vi "Precission to 3 digits.vi"(8 "error in":errorcluster, 11 "Numeric":dbl format="%#_13g") -> (0 "error out":errorcluster, 3 "number":dbl)   [LabVIEW 2015]
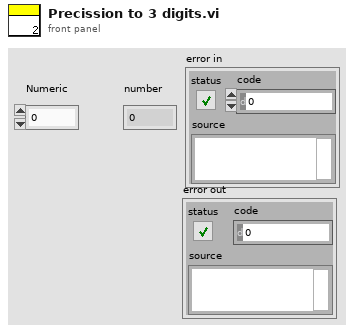
[diagram p1: front panel]
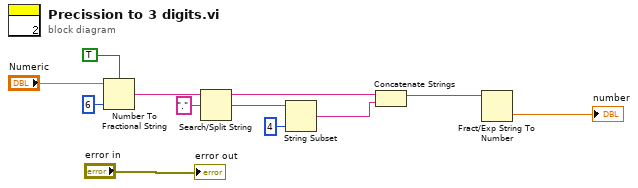
[diagram p0: block diagram]
diagram:
  n1 = Number To Fractional String(use system decimal point (T)=TRUE, number="Numeric", precision (6)=i16 6) -> (F-format string=w5:string)  [unwired: 1 in]
  n2 = Search/Split String(string=w5, search string/char (-)=".") -> (substring before match=w10:string, match + rest of string=w7:string)  [unwired: 1 in, 1 out]
  n3 = String Subset(string=w7, length (rest)=4 ("length (rest)")) -> (substring=w9:string)  [unwired: 1 in]
  n4 = Concatenate Strings(w10, w9) -> (w11:string)
  n5 = Fract/Exp String To Number(string=w11) -> (number=→"number":dbl)  [unwired: 3 in, 1 out]
  "error out" <- "error in"
